vi "InstrumentCalibration - Sensor Setup (SubVI).vi"(8 "error in":errorcluster, 11 "Edit":string[](array[string])) -> (0 "error out":errorcluster)   [LabVIEW 2019]
uses:
  Controls/Sensor Setup - State.ctl
  Controls/Sensor Setup - Data Structure.ctl
  <vilib>/Analysis/NI_AALPro.lvlib
  Controls/FGV States.ctl
  Controls/Calibration - Data Structure.ctl
  Controls/eFGV States.ctl
  <vilib>/Utility/config.llb/NI_LVConfig.lvlib
  <vilib>/Utility/config.llb/Write Key (I32).vi
panel:
  in  "Status":u16(ring) items=["DISABLE", "ACTIVE"]
  in  "Decimal Place":i32=5
  in  "Close":bool
  in  "Load":bool
  in  "Save":bool
  in  "Tab":enum32{"Sensor", "Displacement"}(tab)
  in  "Serial No":string
  in  "Tab 2":enum32{"Direct Factor", "Multiple Point"}(tab)
  in  "Offset":dbl format="%#_5g"
  in  "Max Capacity [EU]":dbl format="%#_5g"
  in  "Maximum Voltage [V]":dbl format="%#_5g"
  in  "Table Control":string[][](table)
  in  "Calibrate":bool
  in  "Sensor Name":string
  in  "Sensor Port":T1(ring)
  in  "Unit":string
  out "Calibrated":dbl
  out "Raw (mV/V)":dbl format="%#_10f"
  out "Disp M":dbl
  in  "Zero":bool
  in  "Unit Disp":string caption="Unit"
  in  "Displacement":dbl
  in  "Calibrate Disp":bool
  out "Motor pulse":u64
  in  "Motor":T2(ring)
  # "1 (Unit) ="
  # "Pulse"
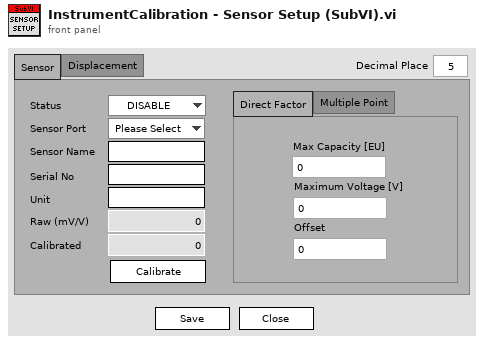
[diagram p1: front panel]
types:
  T1 = enum16{"Please Select", "LC 1", "LC 2", "LC 3", "LC 4", "LC 5", "LC 6", "LC 7", "LC 8", "TD 1", "TD 2", "TD 3", "TD 4", "TD 5", "TD 6", "TD 7", "TD 8", "TD 9", "TD 10", "TD 11", "TD 12"}
  T2 = enum16{"Please Select", "Motor 1", "Motor 2", "Motor 3", "Motor 4", "Motor 5", "Motor 6", "Motor 7", "Motor 8", "Motor 9"}
  T3 = typedef "Sensor Setup - State.ctl" = enum16{"Init", "Idle", "Save", "Close"}
  T4 = enum16{"open", "replace", "create", "open or create", "replace or create", "replace or create with confirmation"}
  T5 = typedef "Sensor Setup - State.ctl" = enum16{"Init", "Idle", "Read", "Calibrate", "Calibrate Disp", "Zeroing", "Zeroing Disp", "Save", "Save Calibration", "Load", "Load Calibration", "Update FGV", "Update GUI", "Close"}
  T6 = typedef "Sensor Setup - Data Structure.ctl" = cluster{"serialno":string, "Name":string, "Channel":string, "Slope":string, "Intercept":string, "Unit":string, "Decimal":string, "New?":bool, "Data":T7, "Port":string[], "IP":string[]}
  T7 = typedef "Calibration - Data Structure.ctl" = cluster{"Timeout":i32, "LC MC":dbl[], "TD MC":dbl[], "Motor Pulse":u64, "Disp M":dbl[], "LC Unit":string[], "Disp Unit":string[], "TD Unit":string[], "LC Name":string[], "TD Name":string[], "Machine":enum16{"Please Select", "Motor 1", "Motor 2", "Motor 3", "Motor 4", "Motor 5", "Motor 6", "Motor 7", "Motor 8", "Motor 9"}, "Sensor Port":enum16{"Please Select", "LC 1", "LC 2", "LC 3", "LC 4", "LC 5", "LC 6", "LC 7", "LC 8", "TD 1", "TD 2", "TD 3", "TD 4", "TD 5", "TD 6", "TD 7", "TD 8", "TD 9", "TD 10", "TD 11", "TD 12"}[]}
  T8 = typedef "FGV States.ctl" = enum16{"Read", "Write"}
  T9 = typedef "eFGV States.ctl" = enum16{"Init", "Read", "Write", "Exit"}
  T10 = cluster{"Zero":bool, "Machine Name":enum16{"Please Select", "Motor 1", "Motor 2", "Motor 3", "Motor 4", "Motor 5", "Motor 6", "Motor 7", "Motor 8", "Motor 9"}}
  T11 = enum16{"Please Select", "LC 1", "LC 2", "LC 3", "LC 4", "LC 5", "LC 6", "LC 7", "LC 8", "TD 1", "TD 2", "TD 3", "TD 4", "TD 5", "TD 6", "TD 7", "TD 8", "TD 9", "TD 10", "TD 11", "TD 12"}[]
  T12 = typedef "NI_LVConfig.lvlib/Config Data RefNum.ctl" = refnum<k1>
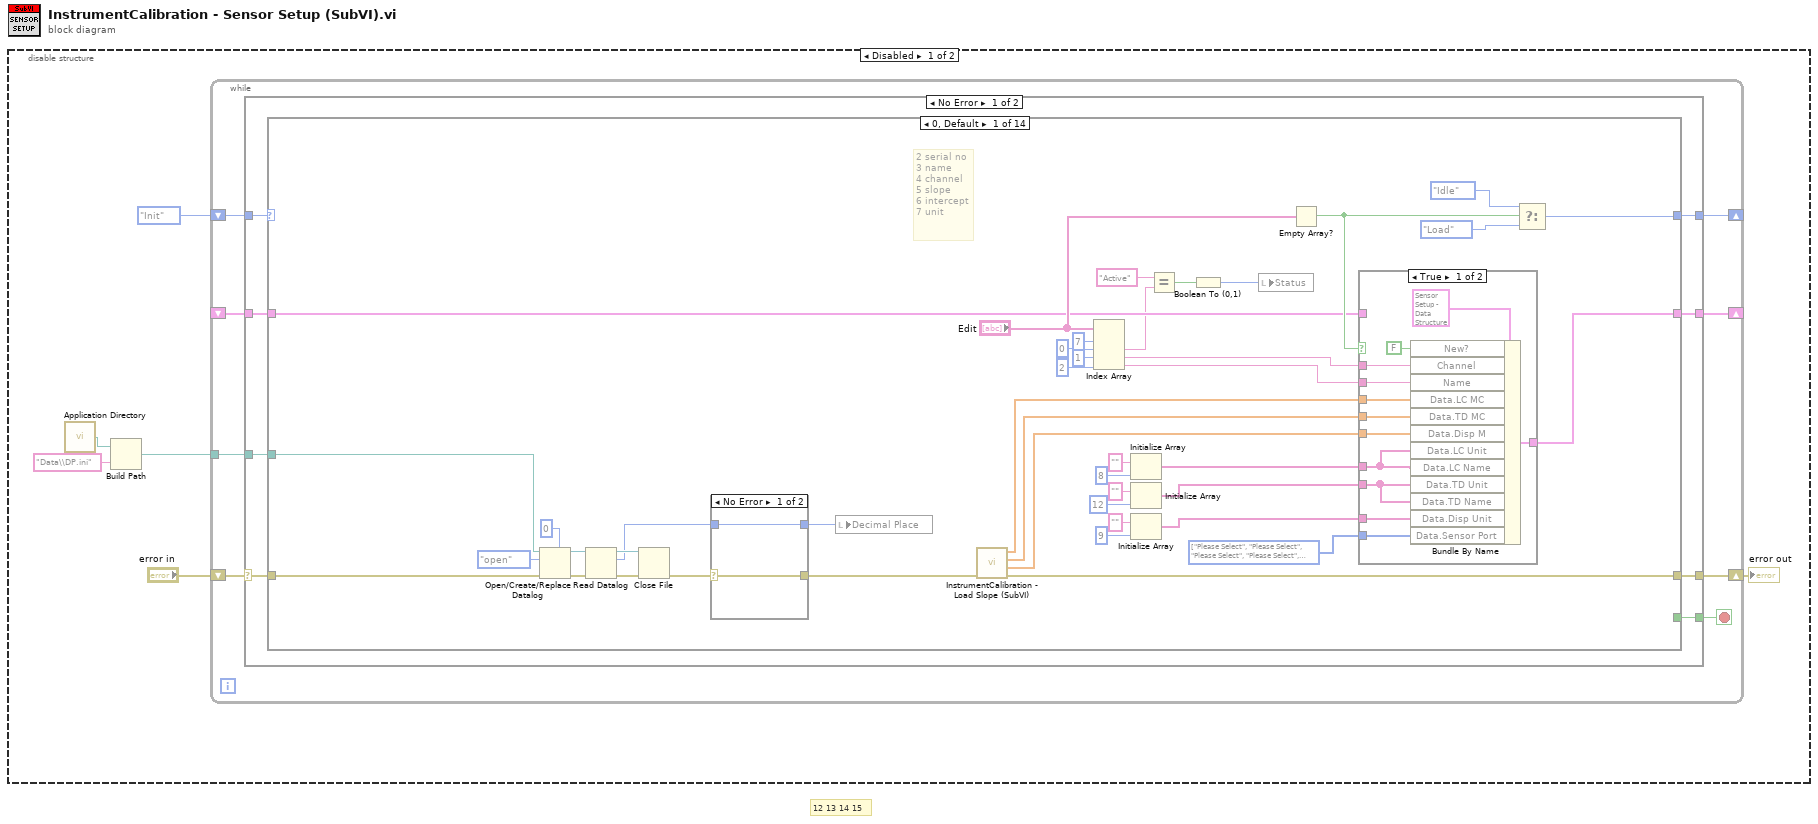
[diagram p0: block diagram]
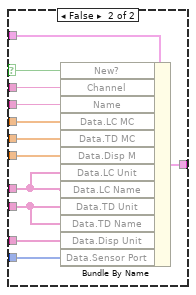
[diagram p2: hidden frame]
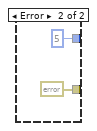
[diagram p3: hidden frame]
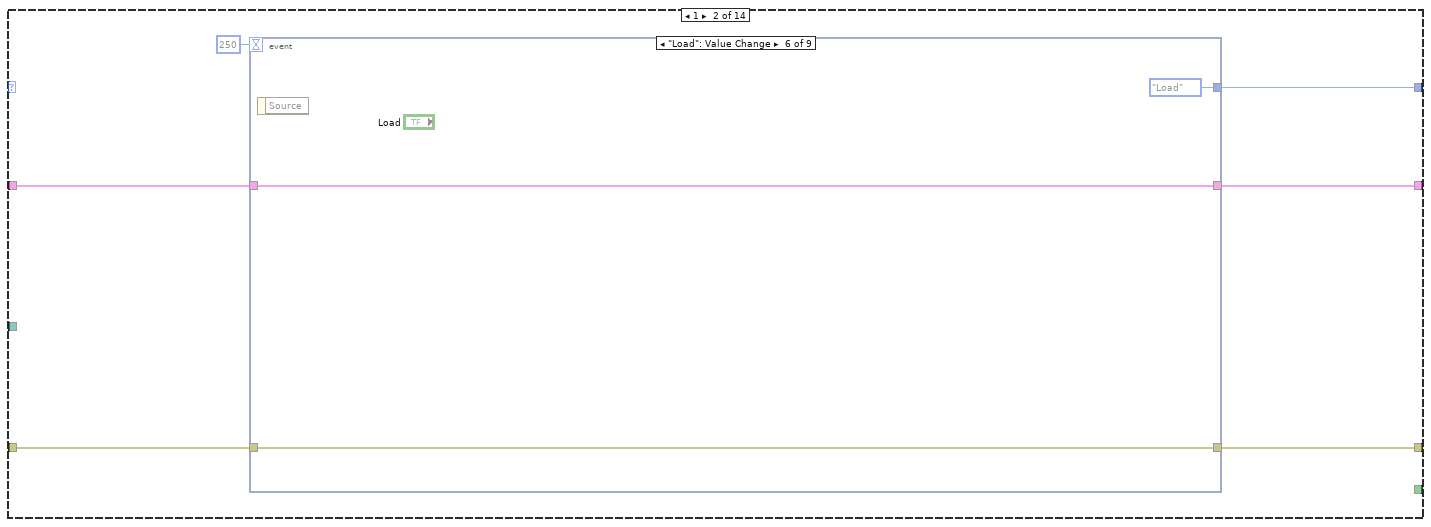
[diagram p4: hidden frame]
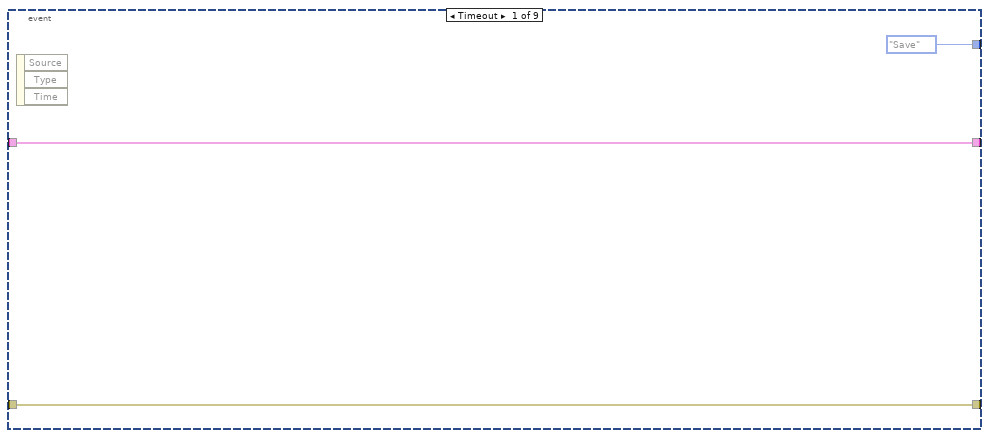
[diagram p5: hidden frame]
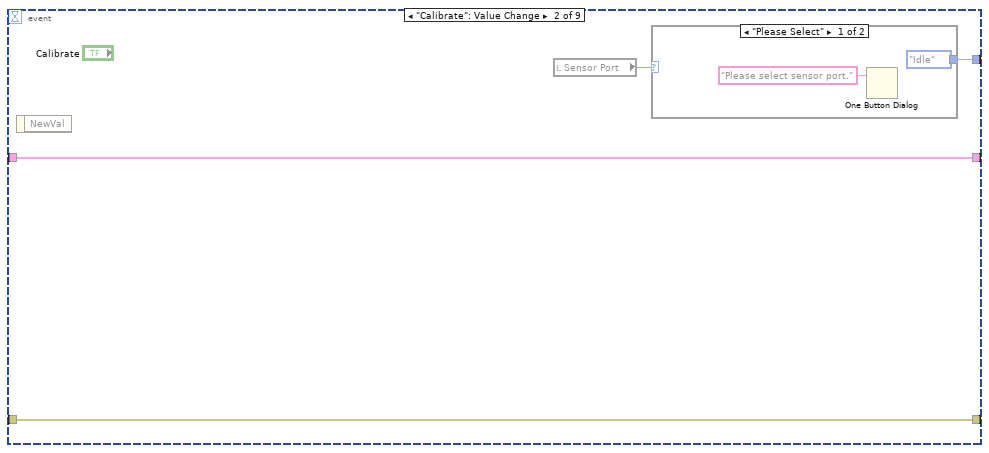
[diagram p6: hidden frame]
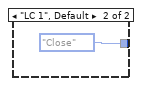
[diagram p7: hidden frame]
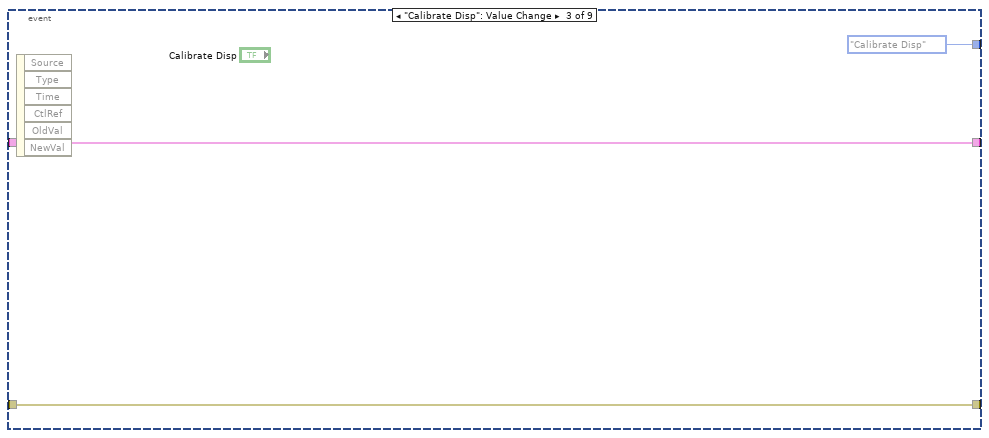
[diagram p8: hidden frame]
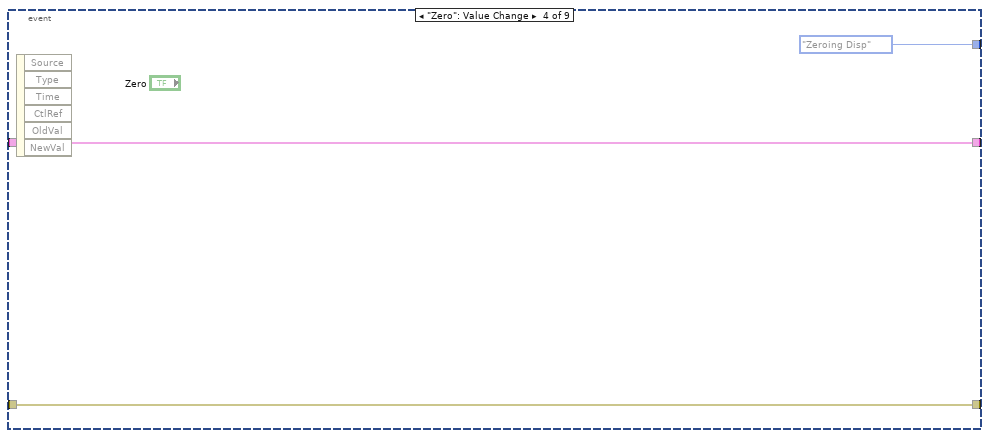
[diagram p9: hidden frame]
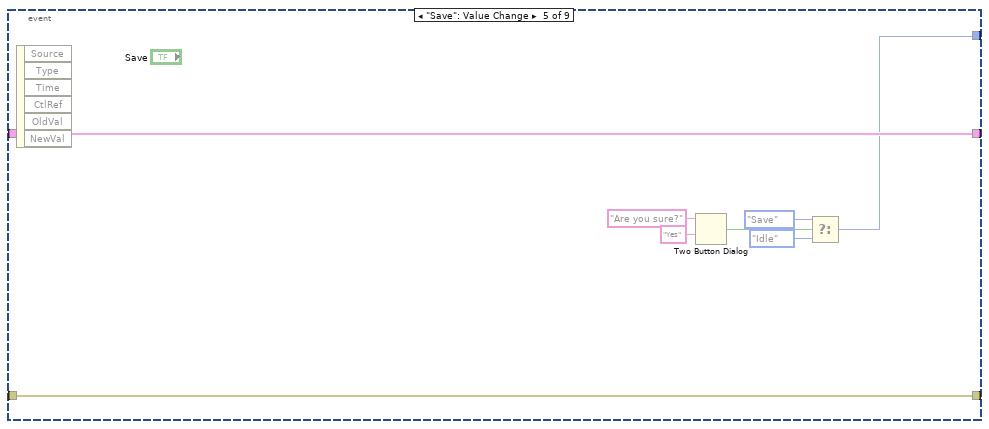
[diagram p10: hidden frame]
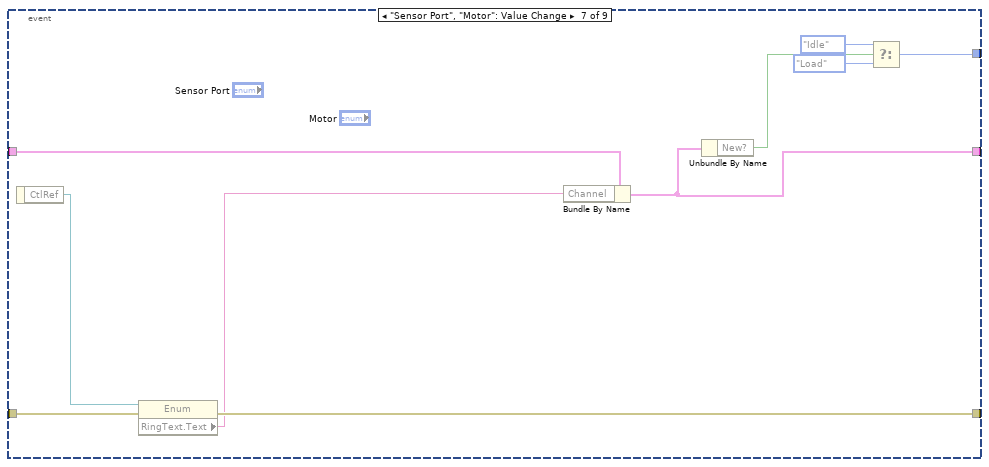
[diagram p11: hidden frame]
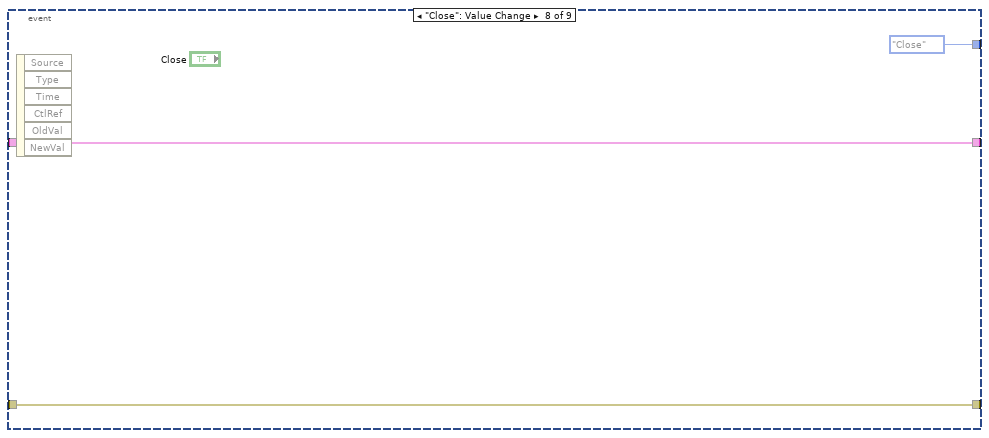
[diagram p12: hidden frame]
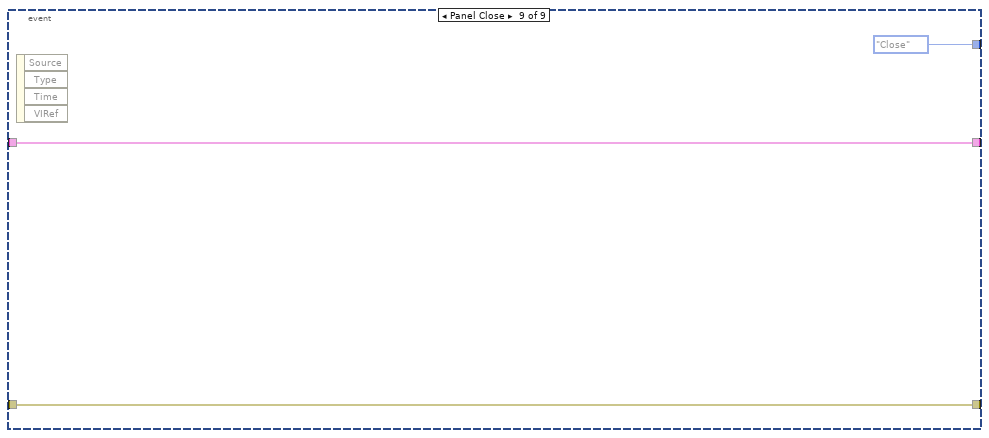
[diagram p13: hidden frame]
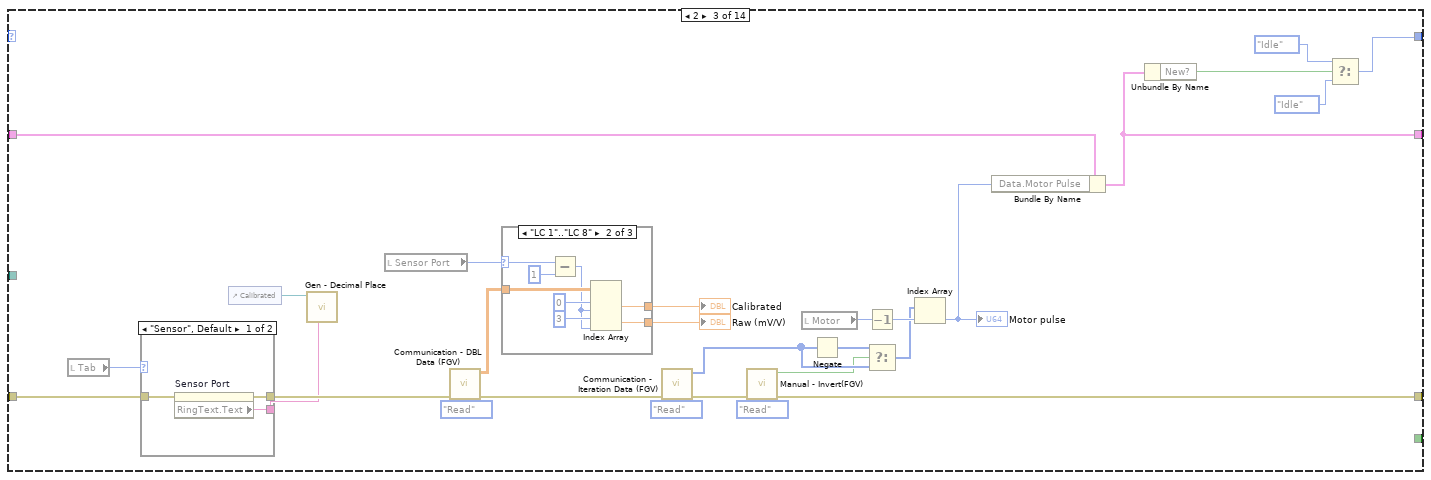
[diagram p14: hidden frame]
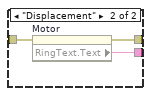
[diagram p15: hidden frame]
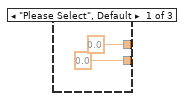
[diagram p16: hidden frame]
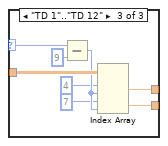
[diagram p17: hidden frame]
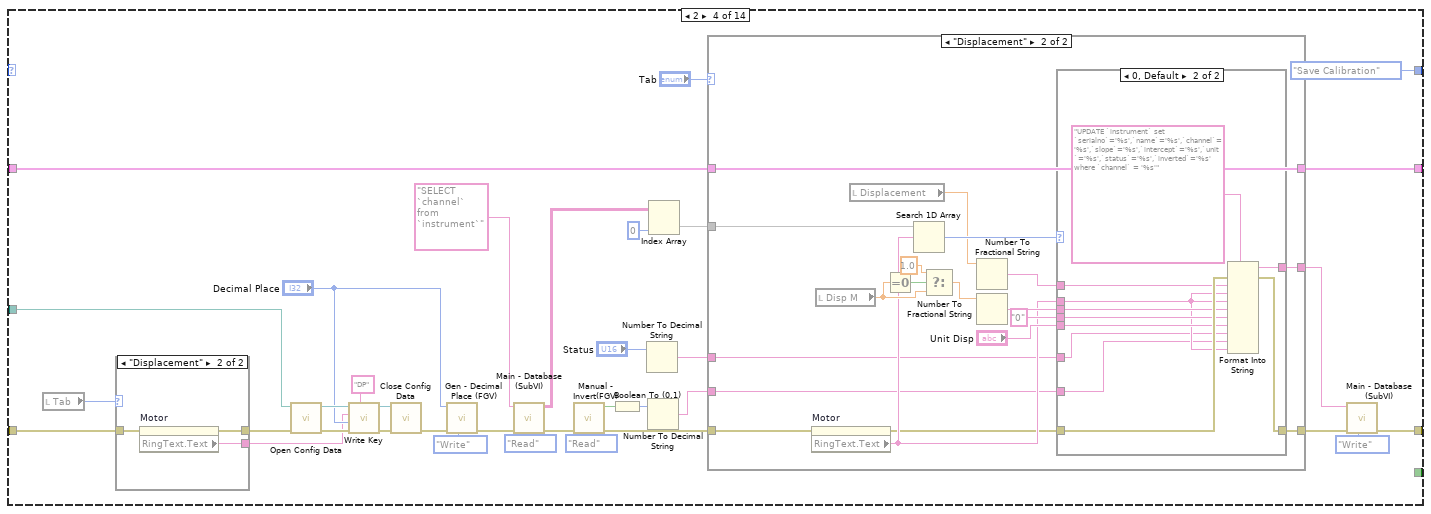
[diagram p18: hidden frame]
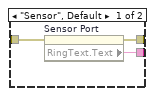
[diagram p19: hidden frame]
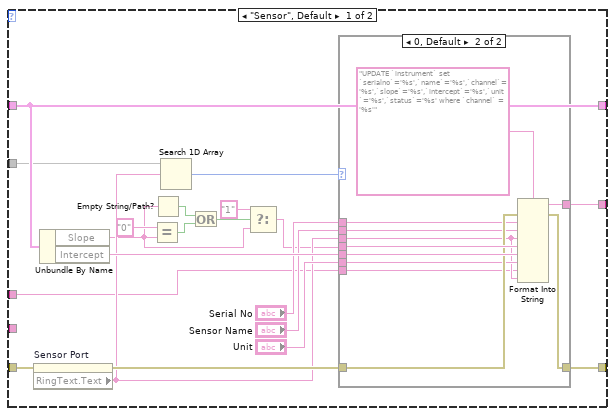
[diagram p20: hidden frame]
diagram:
  # "12 13 14 15"
  n1 = disable-structure shown="Disabled" {
    frame Disabled {
      n2 = call <vilib>:"Application Directory.vi"() -> ("Application Directory"=w3:path)
      n3 = Build Path(base path=w3, name or relative path="Data\\DP.ini") -> (appended path=w1:path)
      n4 = while {
        shift-right: [w13] -> _
        shift-left: Sensor_Setup_-_State."Init" -> [w14]
        shift-right: [w11] -> w4
        shift-left: "error in" -> [w12]
        shift-right: [w9] -> _
        shift-left: _ -> [w8]
        tunnel: w1 -> [w7]
        stop <- w10 stop-if-true
        n5 = case shown="No Error" w12 {
          selector: w12 -> [w19 w673]
          tunnel: w14 -> [w22 w669]
          tunnel: [w21 w669] -> w13
          tunnel: [w20 w672] -> w11
          tunnel: [w18 _] -> w10
          tunnel: [w17 w670] -> w9
          tunnel: w8 -> [w16 w670]
          tunnel: w7 -> [w15 _]
          frame No Error {
            n6 = case shown="0, Default" w22 {
              tunnel: [w60 w97 w159 Sensor_Setup_-_State."Save Calibration" Sensor_Setup_-_State."Load" Sensor_Setup_-_State."Load Calibration" Sensor_Setup_-_State."Update FGV" Sensor_Setup_-_State."Update GUI" Sensor_Setup_-_State."Idle" Sensor_Setup_-_State."Update FGV" Sensor_Setup_-_State."Idle" Sensor_Setup_-_State."Idle" Sensor_Setup_-_State."Close" Sensor_Setup_-_State."Idle"] -> w21
              tunnel: [w30 w99 w151 w225 w319 w367 w480 w526 w544 w570 w649 w652 w656 w659] -> w20
              tunnel: w19 -> [w42 w98 w146 w197 w323 w369 w476 w525 w544 w571 w649 w652 w656 w660]
              tunnel: [_ _ _ _ _ _ _ _ _ _ _ _ TRUE _] -> w18
              tunnel: [w65 w96 w161 w227 w321 w354 w481 w531 w538 w577 w640 w651 w653 w661] -> w17
              tunnel: w16 -> [w32 w95 w163 w228 w322 w353 w483 w531 w541 w565 w639 w651 w653 w661]
              tunnel: w15 -> [w41 _ _ w200 _ _ _ _ _ _ _ _ _ _]
              frame 0, Default {
                w52 = T11 [enum."Please Select", enum."Please Select", enum."Please Select", enum."Please Select", enum."Please Select", enum."Please Select", enum."Please Select", enum."Please Select", enum."Please Select"] items=["Please Select", "LC 1", "LC 2", "LC 3", "LC 4", "LC 5", "LC 6", "LC 7", "LC 8", "TD 1", "TD 2", "TD 3", "TD 4", "TD 5", "TD 6", "TD 7", "TD 8", "TD 9", "TD 10", "TD 11", "TD 12"] ("Sensor Port")
                # "2 serial no\n3 name\n4 channel\n5 slope\n6 intercept\n7 unit"
                n7 = Open/Create/Replace Datalog(5:0, 8:w42, 10:T4."open" ("operation (0:open)"), 11:w41) -> (0:w48:errorcluster, 3:w46:refnum<k1>)  [unwired: 2 in, 1 out]
                n8 = Read Datalog(4:w48, 7:w46) -> (0:w47:errorcluster, 2:w38:i32, 3:w45:refnum<k1>)  [unwired: 1 in]
                n9 = Close File(refnum=w45, error in=w47) -> (error out=w40:errorcluster)  [unwired: 1 out]
                n10 = case shown="No Error" w40 {
                  selector: w40 -> [w90 _]
                  tunnel: [w91 5] -> w39
                  tunnel: w38 -> [w91 _]
                  tunnel: [w90 errorcluster {"status"=FALSE, "code"=0, "source"=""} ("error IO")] -> w31
                  frame No Error {
                  }
                  frame Error {
                  }
                }
                n11 = local write "Decimal Place"(w39) -> ()
                n12 = call "InstrumentCalibration - Load Slope (SubVI).vi"("error in (no error)"=w31) -> ("error out"=w30:errorcluster, "Motor M"=w27:dbl[], "TD MC"=w28:dbl[], "LC MC"=w29:dbl[])  [unwired: 7 in]
                n13 = Index Array(array="Edit", index #1=7 ("index"), index #2=0 ("index"), index #3=1 ("index"), index #4=2 ("index")) -> (element #2=w26:string, element #3=w64:string, element #4=w63:string)  [unwired: 1 out]
                n14 = Initialize Array("" ("element"), 8 ("dimension size")) -> (w51:string[])
                n15 = Initialize Array("" ("element"), 12 ("dimension size")) -> (w50:string[])
                n16 = Initialize Array("" ("element"), 9 ("dimension size")) -> (w49:string[])
                n17 = Equal?(x="Active", y=w26) -> (x = y?=w24:bool)
                n18 = Boolean To (0,1)(Boolean=w24) -> (0, 1=w23:i16)
                n19 = local write "Status"(w23) -> ()
                n20 = Empty Array?(array="Edit") -> (empty?=w33:bool)
                n21 = case shown="True" w33 {
                  selector: w33 -> [_ w81]
                  tunnel: [w76 w89] -> w65
                  tunnel: w64 -> [w75 w88]
                  tunnel: w63 -> [w74 w87]
                  tunnel: w52 -> [w73 w86]
                  tunnel: w29 -> [w72 w85]
                  tunnel: w28 -> [w71 w84]
                  tunnel: w27 -> [w70 w83]
                  tunnel: w51 -> [w68 w80]
                  tunnel: w50 -> [w67 w79]
                  tunnel: w49 -> [w69 w82]
                  tunnel: w32 -> [_ w78]
                  frame True {
                    n22 = Bundle By Name(cluster=T6 {"serialno"="", "Name"="", "Channel"="", "Slope"="", "Intercept"="", "Unit"="", "Decimal"="", "New?"=FALSE, "Data"={"Timeout"=-1, "LC MC"=[], "TD MC"=[], "Motor Pulse"=0, "Disp M"=[], "LC Unit"=[], "Disp Unit"=[], "TD Unit"=[], "LC Name"=[], "TD Name"=[], "Machine"=enum."Please Select", "Sensor Port"=[]}, "Port"=[], "IP"=[]}, "New?"=FALSE, "Channel"=w75, "Name"=w74, "Data.LC MC"=w72, "Data.TD MC"=w71, "Data.Disp M"=w70, "Data.LC Unit"=w68, "Data.LC Name"=w68, "Data.TD Unit"=w67, "Data.TD Name"=w67, "Data.Disp Unit"=w69, "Data.Sensor Port"=w73) -> (w76:T6)
                  }
                  frame False {
                    n23 = Bundle By Name(cluster=w78, "New?"=w81, "Channel"=w88, "Name"=w87, "Data.LC MC"=w85, "Data.TD MC"=w84, "Data.Disp M"=w83, "Data.LC Unit"=w80, "Data.LC Name"=w80, "Data.TD Unit"=w79, "Data.TD Name"=w79, "Data.Disp Unit"=w82, "Data.Sensor Port"=w86) -> (w89:T6)
                  }
                }
                n24 = Select(t=Sensor_Setup_-_State."Idle", s=w33, f=Sensor_Setup_-_State."Load") -> (s? t:f=w60:u16)
              }
              frame 1 {
                n25 = event shown="[5] \"Load\": Value Change" {
                  selector: _ -> [_ _ _ _ _ _ _ _ _]
                  dyn-events: _ -> [_ _ _ _ _ _ _ _ _]
                  timeout: 250 -> [_ _ _ _ _ _ _ _ _]
                  tunnel: [w102 w106 w112 w115 w123 w126 w134 w139 w142] -> w99
                  tunnel: w98 -> [w102 w106 w112 w115 w123 w126 w133 w139 w142]
                  tunnel: [Sensor_Setup_-_State."Save" w105 Sensor_Setup_-_State."Calibrate Disp" Sensor_Setup_-_State."Zeroing Disp" w117 Sensor_Setup_-_State."Load" w128 Sensor_Setup_-_State."Close" Sensor_Setup_-_State."Close"] -> w97
                  tunnel: [w100 w104 w110 w113 w122 w124 w131 w138 w141] -> w96
                  tunnel: w95 -> [w100 w104 w110 w113 w122 w124 w136 w138 w141]
                  event Timeout {
                    n26 = event-data() -> ()  [unwired: 1 in, 3 out]
                  }
                  event "Calibrate": Value Change {
                    n27 = event-data() -> ()  [unwired: 1 in, 1 out]
                    n28 = local read "Sensor Port"() -> (w103:T1)
                    n29 = case shown="\"Please Select\"" w103 {
                      tunnel: [Sensor_Setup_-_State."Idle" Sensor_Setup_-_State."Close"] -> w105
                      frame "Please Select" {
                        n30 = One Button Dialog(message="Please select sensor port.") -> ()  [unwired: 1 in, 1 out]
                      }
                      frame "LC 1", Default {
                      }
                    }
                  }
                  event "Calibrate Disp": Value Change {
                    n31 = event-data() -> ()  [unwired: 1 in, 6 out]
                  }
                  event "Zero": Value Change {
                    n32 = event-data() -> ()  [unwired: 1 in, 6 out]
                  }
                  event "Save": Value Change {
                    n33 = event-data() -> ()  [unwired: 1 in, 6 out]
                    n34 = Two Button Dialog(message="Are you sure?", 2:"Yes" ("T button name (\"OK\")")) -> (T button?=w119:bool)  [unwired: 1 in]
                    n35 = Select(t=Sensor_Setup_-_State."Save", s=w119, f=Sensor_Setup_-_State."Idle") -> (s? t:f=w117:T3)
                  }
                  event "Load": Value Change {
                    n36 = event-data() -> ()  [unwired: 1 in, 1 out]
                  }
                  event "Sensor Port", "Motor": Value Change {
                    n37 = event-data() -> ("CtlRef"=w135:refnum<vi>)  [unwired: 1 in]
                    n38 = property class="Enum"(reference=w135, error in=w133) -> (error out=w134:errorcluster, "RingText.Text"=w132:string)  [unwired: 1 out]
                    n39 = Bundle By Name(cluster=w136, "Channel"=w132) -> (w131:T6)
                    n40 = Unbundle By Name(w131) -> ("New?"=w130:bool)
                    n41 = Select(t=Sensor_Setup_-_State."Idle", s=w130, f=Sensor_Setup_-_State."Load") -> (s? t:f=w128:u16)
                  }
                  event "Close": Value Change {
                    n42 = event-data() -> ()  [unwired: 1 in, 6 out]
                  }
                  event Panel Close {
                    n43 = event-data() -> ()  [unwired: 1 in, 4 out]
                  }
                }
              }
              frame 2 {
                n44 = local read "Tab"() -> (w147:enum32{"Sensor", "Displacement"})
                n45 = case shown="\"Sensor\", Default" w147 {
                  tunnel: [w172 w176] -> w145
                  tunnel: w146 -> [w173 w175]
                  tunnel: [w171 w174] -> w144
                  frame "Sensor", Default {
                    n46 = property on="Sensor Port" class="Enum (strict)"(error in=w173) -> (error out=w172:errorcluster, "RingText.Text"=w171:string)  [unwired: 1 in, 1 out]
                  }
                  frame "Displacement" {
                    n47 = property on="Motor" class="Enum (strict)"(error in=w175) -> (error out=w176:errorcluster, "RingText.Text"=w174:string)  [unwired: 1 in, 1 out]
                  }
                }
                n48 = control-ref of="Calibrated"() -> (w143:refnum<vi>)
                n49 = call "Gen - Decimal Place.vi"(7:w144, "DigNum Refnum"=w143) -> ()  [unwired: 10 in]
                n50 = local read "Sensor Port"() -> (w148:T1)
                n51 = call "Communication - DBL Data (FGV).vi"("Action"=FGV_States."Read", "error in (no error)"=w145) -> ("error out"=w152:errorcluster, "DBL SV Out"=w169:dbl[][])  [unwired: 8 in]
                n52 = case shown="\"LC 1\"..\"LC 8\"" w148 {
                  selector: w148 -> [_ w181 w191]
                  tunnel: w169 -> [_ w186 w194]
                  tunnel: [0.0 ("shared variable refnum in") w185 w193] -> w168
                  tunnel: [0.0 ("shared variable refnum in") w184 w192] -> w167
                  frame "Please Select", Default {
                  }
                  frame "LC 1".."LC 8" {
                    n53 = Subtract(x=w181, y=1 ("disabled index (col)")) -> (x-y=w180:i32)
                    n54 = Index Array(array=w186, index (row) #1=0 ("disabled index (col)"), index (col) #1=w180, index (row) #2=3 ("index (col)"), index (col) #2=w180) -> (element #1=w185:dbl, element #2=w184:dbl)
                  }
                  frame "TD 1".."TD 12" {
                    n55 = Subtract(x=w191, y=9 ("disabled index (col)")) -> (x-y=w189:i32)
                    n56 = Index Array(array=w194, index (row) #1=4 ("disabled index (col)"), index (col) #1=w189, index (row) #2=7 ("index (col)"), index (col) #2=w189) -> (element #1=w193:dbl, element #2=w192:dbl)
                  }
                }
                "Raw (mV/V)" <- w167
                "Calibrated" <- w168
                n57 = call "Communication - Iteration Data (FGV).vi"("Action"=FGV_States."Read", "error in (no error)"=w152) -> ("error out"=w150:errorcluster, "Iteration SV Out"=w155:i64[])  [unwired: 8 in]
                n58 = call "Manual - Invert(FGV).vi"("Action"=FGV_States."Read", "error in (no error)"=w150) -> ("error out"=w151:errorcluster, "invert out"=w149:bool)  [unwired: 8 in]
                n59 = local read "Motor"() -> (w165:T2)
                n60 = Negate(x=w155) -> (-x=w156:i64[])
                n61 = Decrement(x=w165) -> (x-1=w166:T2)
                n62 = Select(t=w156, s=w149, f=w155) -> (s? t:f=w154:i64[])
                n63 = Index Array(array=w154, index=w166) -> (element=w162:i64)
                "Motor pulse" <- w162
                n64 = Bundle By Name(cluster=w163, "Data.Motor Pulse"=w162) -> (w161:T6)
                n65 = Unbundle By Name(w161) -> ("New?"=w160:bool)
                n66 = Select(t=Sensor_Setup_-_State."Idle", s=w160, f=Sensor_Setup_-_State."Idle") -> (s? t:f=w159:T3)
              }
              frame 2 {
                n67 = local read "Tab"() -> (w195:enum32{"Sensor", "Displacement"})
                n68 = case shown="\"Displacement\"" w195 {
                  tunnel: [w231 w235] -> w198
                  tunnel: w197 -> [w232 w234]
                  tunnel: [w230 w233] -> w196
                  frame "Sensor", Default {
                    n69 = property on="Sensor Port" class="Enum (strict)"(error in=w232) -> (error out=w231:errorcluster, "RingText.Text"=w230:string)  [unwired: 1 in, 1 out]
                  }
                  frame "Displacement" {
                    n70 = property on="Motor" class="Enum (strict)"(error in=w234) -> (error out=w235:errorcluster, "RingText.Text"=w233:string)  [unwired: 1 in, 1 out]
                  }
                }
                n71 = call <vilib>:"Open Config Data.vi"("error in (no error)"=w198, "configuration file path"=w200) -> ("error out"=w205:errorcluster, "refnum"=w203:T12)  [unwired: 7 in, 1 out]
                n72 = call-poly <vilib>:"Write Key.vi"("section"="DP", "error in (no error)"=w205, "value"="Decimal Place", "key"=w196, "refnum"=w203) -> ("error out"=w206:errorcluster, "refnum out"=w204:T12)  [unwired: 4 in, 1 out]
                n73 = call <vilib>:"Close Config Data.vi"("error in (no error)"=w206, "refnum"=w204) -> ("error out"=w201:errorcluster)  [unwired: 8 in, 1 out]
                n74 = call "Gen - Decimal Place (FGV).vi"("Action"=FGV_States."Write", "error In"=w201, "Ch1"="Decimal Place") -> ("error out"=w210:errorcluster)  [unwired: 6 in, 2 out]
                n75 = call "Main - Database (SubVI).vi"("Enum"=FGV_States."Read", "error in (no error)"=w210, "SQL query"="SELECT `channel` from `instrument`") -> ("error out"=w215:errorcluster, "data"=w219:string[][])  [unwired: 7 in]
                n76 = call "Manual - Invert(FGV).vi"("Action"=FGV_States."Read", "error in (no error)"=w215) -> ("error out"=w214:errorcluster, "invert out"=w213:bool)  [unwired: 8 in]
                n77 = Boolean To (0,1)(Boolean=w213) -> (0, 1=w209:i16)
                n78 = Number To Decimal String(number="Status") -> (decimal integer string=w207:string)  [unwired: 1 in]
                n79 = Number To Decimal String(number=w209) -> (decimal integer string=w212:string)  [unwired: 1 in]
                n80 = Index Array(array=w219, index (col)=0 ("disabled index (col)")) -> (element=w218:string[])  [unwired: 1 in]
                n81 = case shown="\"Displacement\"" "Tab" {
                  tunnel: w228 -> [w255 w296]
                  tunnel: [w255 w296] -> w227
                  tunnel: w214 -> [w252 w295]
                  tunnel: [w248 w291] -> w223
                  tunnel: [w247 w290] -> w222
                  tunnel: w218 -> [w246 w289]
                  tunnel: w212 -> [_ w279]
                  tunnel: w207 -> [w236 w278]
                  frame "Sensor", Default {
                    n82 = property on="Sensor Port" class="Enum (strict)"(error in=w252) -> (error out=w253:errorcluster, "RingText.Text"=w245:string)  [unwired: 1 in, 1 out]
                    n83 = Unbundle By Name(w255) -> ("Slope"=w239:string, "Intercept"=w254:string)
                    n84 = Equal?(x="0", y=w239) -> (x = y?=w241:bool)
                    n85 = Empty String/Path?(string/path=w239) -> (empty?=w242:bool)
                    n86 = Search 1D Array(1D array=w246, element=w245) -> (index of element=w244:i32)  [unwired: 1 in]
                    n87 = Or(x=w242, y=w241) -> (x .or. y?=w240:bool)
                    n88 = Select(t="1", s=w240, f=w239) -> (s? t:f=w237:string)
                    n89 = case shown="0, Default" w244 {
                      tunnel: w237 -> [w265 w277]
                      tunnel: w254 -> [w264 w276]
                      tunnel: w253 -> [w263 w275]
                      tunnel: "Unit" -> [w262 w274]
                      tunnel: "Serial No" -> [w261 w273]
                      tunnel: "Sensor Name" -> [w260 w272]
                      tunnel: w245 -> [w259 w268]
                      tunnel: [w258 w271] -> w248
                      tunnel: [w257 w270] -> w247
                      tunnel: w236 -> [w256 w267]
                      frame -1 {
                        n90 = Format Into String(format string="INSERT INTO `instrument`  (`serialno`,`name`,`channel`,`slope`,`intercept`,`unit`,`status`) VALUES ('%s','%s','%s','%s','%s','%s','%s')" ("SQL query"), error in=w263, w261, w260, w259, w265, w264, w262, w256) -> (resulting string=w257:string, error out=w258:errorcluster)  [unwired: 1 in]
                      }
                      frame 0, Default {
                        n91 = Format Into String(format string="UPDATE `instrument` set `serialno`='%s',`name`='%s',`channel`='%s',`slope`='%s',`intercept`='%s',`unit`='%s',`status`='%s' where `channel` = '%s'" ("SQL query"), error in=w275, w273, w272, w268, w277, w276, w274, w267, w268) -> (resulting string=w270:string, error out=w271:errorcluster)  [unwired: 1 in]
                      }
                    }
                  }
                  frame "Displacement" {
                    n92 = property on="Motor" class="Enum (strict)"(error in=w295) -> (error out=w280:errorcluster, "RingText.Text"=w281:string)  [unwired: 1 in, 1 out]
                    n93 = local read "Disp M"() -> (w285:dbl)
                    n94 = local read "Displacement"() -> (w283:dbl)
                    n95 = Equal To 0?(x=w285) -> (x = 0?=w287:bool)
                    n96 = Search 1D Array(1D array=w289, element=w281) -> (index of element=w288:i32)  [unwired: 1 in]
                    n97 = Select(t=1.0, s=w287, f=w285) -> (s? t:f=w284:dbl)
                    n98 = Number To Fractional String(number=w283) -> (F-format string=w282:string)  [unwired: 3 in]
                    n99 = Number To Fractional String(number=w284) -> (F-format string=w292:string)  [unwired: 3 in]
                    n100 = case shown="0, Default" w288 {
                      tunnel: w280 -> [w306 w317]
                      tunnel: w281 -> [w300 w310]
                      tunnel: "Unit Disp" -> [w305 w316]
                      tunnel: "0" -> [w304 w315]
                      tunnel: w292 -> [w303 w314]
                      tunnel: [w302 w313] -> w291
                      tunnel: [w301 w312] -> w290
                      tunnel: w282 -> [w299 w311]
                      tunnel: w279 -> [w297 w309]
                      tunnel: w278 -> [w298 w308]
                      frame -1 {
                        n101 = Format Into String(format string="INSERT INTO `instrument`  (`serialno`,`name`,`channel`,`slope`,`intercept`,`unit`,`status`,`inverted`) VALUES ('%s','%s','%s','%s','%s','%s','%s','%s')" ("SQL query"), error in=w306, w299, w300, w300, w303, w304, w305, w298, w297) -> (resulting string=w301:string, error out=w302:errorcluster)  [unwired: 1 in]
                      }
                      frame 0, Default {
                        n102 = Format Into String(format string="UPDATE `instrument` set `serialno`='%s',`name`='%s',`channel`='%s',`slope`='%s',`intercept`='%s',`unit`='%s',`status`='%s',`inverted`='%s' where `channel` = '%s'" ("SQL query"), error in=w317, w311, w310, w310, w314, w315, w316, w308, w309, w310) -> (resulting string=w312:string, error out=w313:errorcluster)  [unwired: 1 in]
                      }
                    }
                  }
                }
                n103 = call "Main - Database (SubVI).vi"("Enum"=FGV_States."Write", "error in (no error)"=w223, "SQL query"=w222) -> ("error out"=w225:errorcluster)  [unwired: 7 in, 1 out]
              }
              frame 3 {
                n104 = local read "Tab"() -> (w320:enum32{"Sensor", "Displacement"})
                n105 = case shown="\"Sensor\"" w320 {
                  tunnel: w322 -> [w346 w352]
                  tunnel: [w346 w352] -> w321
                  tunnel: w323 -> [w344 w351]
                  tunnel: [w339 w351] -> w319
                  frame "Sensor" {
                    n106 = local read "Table Control"() -> (w325:string[][])
                    n107 = for {
                      tunnel: w325 -> [w347] mode=indexing
                      tunnel: [w348] -> w327 mode=indexing
                      n108 = Array To Spreadsheet String(delimiter (Tab)=",,", array=w347, 3:"" ("format string")) -> (spreadsheet string=w348:string)
                    }
                    n109 = Array To Spreadsheet String(delimiter (Tab)="||", array=w327, 3:"" ("format string")) -> (spreadsheet string=w326:string)
                    n110 = local read "Maximum Voltage [V]"() -> (w332:dbl)
                    n111 = local read "Max Capacity [EU]"() -> (w333:dbl)
                    n112 = property on="Sensor Port" class="Enum (strict)"(error in=w344) -> (error out=w345:errorcluster, "RingText.Text"=w343:string)  [unwired: 1 in, 1 out]
                    n113 = local read "Tab 2"() -> (w337:enum32{"Direct Factor", "Multiple Point"})
                    n114 = Number To Fractional String(number=w333, precision (6)=i16 6) -> (F-format string=w331:string)  [unwired: 2 in]
                    n115 = Number To Fractional String(number=w332, precision (6)=i16 6) -> (F-format string=w330:string)  [unwired: 2 in]
                    n116 = Number To Decimal String(number=w337) -> (decimal integer string=w336:string)  [unwired: 1 in]
                    n117 = Format Into String(format string="UPDATE `instrument` set `tab`='%s',`max_cap`='%s',`max_v`='%s',`multipoint`='%s'  where `channel` = '%s'" ("SQL query"), error in=w345, w336, w331, w330, w326, w343) -> (resulting string=w338:string, error out=w340:errorcluster)  [unwired: 1 in]
                    n118 = call "Main - Database (SubVI).vi"("Enum"=FGV_States."Write", "error in (no error)"=w340, "SQL query"=w338) -> ("error out"=w339:errorcluster)  [unwired: 7 in, 1 out]
                  }
                  frame "Displacement", Default {
                  }
                }
              }
              frame 1 {
                n119 = Unbundle By Name(w353) -> ("Channel"=w366:string)
                n120 = Search and Replace String(input string=w366, search string="Motor", error in=w369) -> (number of replacements=w368:i32, error out=w370:errorcluster)  [unwired: 5 in, 2 out]
                n121 = case shown="..0" w368 {
                  tunnel: [w468 w473] -> w364
                  tunnel: w370 -> [w467 w474]
                  tunnel: w366 -> [w464 w469]
                  tunnel: [w464 w469] -> w358
                  tunnel: [enum32{"Sensor", "Displacement"}."Sensor" ("Tab") enum32{"Sensor", "Displacement"}."Displacement" ("Tab")] -> w356
                  frame ..0 {
                    n122 = property on="Sensor Port" class="Enum (strict)"(error in=w467) -> (error out=w468:errorcluster, "Strings []"=w466:string[])  [unwired: 1 in, 1 out]
                    n123 = Search 1D Array(1D array=w466, element=w464) -> (index of element=w465:i32)  [unwired: 1 in]
                    n124 = local write "Sensor Port"(w465) -> ()
                  }
                  frame 1.. {
                    n125 = property on="Motor" class="Enum (strict)"(error in=w474) -> (error out=w473:errorcluster, "Strings []"=w471:string[])  [unwired: 1 in, 1 out]
                    n126 = Search 1D Array(1D array=w471, element=w469) -> (index of element=w472:i32)  [unwired: 1 in]
                    n127 = local write "Motor"(w472) -> ()
                  }
                }
                n128 = Format Into String(format string="SELECT * from `instrument` where `channel` ='%s'" ("SQL query"), error in=w364, w358) -> (resulting string=w361:string, error out=w363:errorcluster)  [unwired: 1 in]
                n129 = local write "Tab"(w356) -> ()
                n130 = call "Main - Database (SubVI).vi"("Enum"=FGV_States."Read", "error in (no error)"=w363, "SQL query"=w361) -> ("error out"=w355:errorcluster, "data"=w360:string[][])  [unwired: 7 in]
                n131 = Index Array(array=w360, index (row)=0) -> (element=w357:string[])  [unwired: 1 in]
                n132 = case shown="\"Sensor\", Default" w356 {
                  tunnel: w357 -> [w397 w462]
                  tunnel: [w388 w461] -> w367
                  tunnel: w355 -> [w389 w461]
                  tunnel: w353 -> [w393 w454]
                  tunnel: w353 -> [w390 w453]
                  tunnel: [w387 w452] -> w354
                  frame "Sensor", Default {
                    n133 = Index Array(array=w397, index #1=2 ("index"), index #2=3 ("index"), index #3=5 ("index"), index #4=6 ("index"), index #5=7 ("index"), index #6=11 ("index")) -> (element #1=w386:string, element #2=w385:string, element #3=w382:string, element #4=w381:string, element #5=w384:string, element #6=w374:string)
                    n134 = local read "Sensor Port"() -> (w383:T1)
                    n135 = Decimal String To Number(string=w374) -> (number=w373:i32)  [unwired: 2 in, 1 out]
                    n136 = Fract/Exp String To Number(string=w382) -> (number=w380:dbl)  [unwired: 3 in, 1 out]
                    n137 = Fract/Exp String To Number(string=w381) -> (number=w379:dbl)  [unwired: 3 in, 1 out]
                    n138 = case shown="\"TD 1\"..\"TD 12\"" w383 {
                      selector: w383 -> [_ w416 w438]
                      tunnel: w393 -> [w402 w422 w443]
                      tunnel: w390 -> [_ w421 w442]
                      tunnel: w389 -> [w398 w420 w441]
                      tunnel: [w398 w420 w441] -> w388
                      tunnel: [w402 w419 w440] -> w387
                      tunnel: w386 -> [_ w405 w423]
                      tunnel: w385 -> [_ w404 w428]
                      tunnel: w384 -> [_ w403 w429]
                      tunnel: w380 -> [_ w408 w436]
                      tunnel: w379 -> [_ w407 w435]
                      tunnel: ["" ("Value") w405 w423] -> w378
                      tunnel: ["" ("Value") w404 w428] -> w377
                      tunnel: ["" ("Value") w403 w429] -> w376
                      frame "Please Select", Default {
                      }
                      frame "LC 1".."LC 8" {
                        n139 = Decrement(x=w416) -> (x-1=w411:T1)
                        n140 = Unbundle By Name(w421) -> ("Data.LC MC"=w418:dbl[], "Data.LC Unit"=w413:string[], "Data.LC Name"=w410:string[])
                        n141 = Multiply(x=w411, y=2) -> (x*y=w415:i32)
                        n142 = Increment(x=w415) -> (x+1=w414:i32)
                        n143 = Replace Array Subset(array=w418, new element #1=w408, index #1=w415, new element #2=w407, index #2=w414) -> (w406:dbl[])
                        n144 = Replace Array Subset(array=w413, new element=w403, index=w411) -> (w412:string[])
                        n145 = Replace Array Subset(array=w410, new element=w404, index=w411) -> (w409:string[])
                        n146 = Bundle By Name(cluster=w422, "Data.LC MC"=w406, "Data.LC Unit"=w412, "Data.LC Name"=w409, "serialno"=w405) -> (w419:T6)
                      }
                      frame "TD 1".."TD 12" {
                        n147 = Unbundle By Name(w442) -> ("Data.TD MC"=w439:dbl[], "Data.TD Unit"=w433:string[], "Data.TD Name"=w432:string[])
                        n148 = Subtract(x=w438, y=9) -> (x-y=w424:i32)
                        n149 = Multiply(x=w424, y=2) -> (x*y=w426:i32)
                        n150 = Increment(x=w426) -> (x+1=w425:i32)
                        n151 = Replace Array Subset(array=w439, new element #1=w436, index #1=w426, new element #2=w435, index #2=w425) -> (w434:dbl[])
                        n152 = Replace Array Subset(array=w433, new element=w429, index=w424) -> (w430:string[])
                        n153 = Replace Array Subset(array=w432, new element=w428, index=w424) -> (w431:string[])
                        n154 = Bundle By Name(cluster=w443, "Data.TD MC"=w434, "Data.TD Unit"=w430, "Data.TD Name"=w431, "serialno"=w423) -> (w440:T6)
                      }
                    }
                    n155 = local write "Status"(w373) -> ()
                    n156 = local write "Serial No"(w378) -> ()
                    n157 = local write "Sensor Name"(w377) -> ()
                    n158 = local write "Unit"(w376) -> ()
                  }
                  frame "Displacement" {
                    n159 = Index Array(array=w462, index #1=2 ("index"), index #2=5 ("index"), index #3=7 ("index")) -> (element #1=w457:string, element #2=w455:string, element #3=w445:string)
                    n160 = Unbundle By Name(w453) -> ("Data.Disp M"=w451:dbl[], "Data.Disp Unit"=w447:string[])
                    n161 = local read "Motor"() -> (w450:T2)
                    n162 = Fract/Exp String To Number(string=w457) -> (number=w456:dbl)  [unwired: 3 in, 1 out]
                    n163 = Fract/Exp String To Number(string=w455) -> (number=w449:dbl)  [unwired: 3 in, 1 out]
                    n164 = Decrement(x=w450) -> (x-1=w446:T2)
                    n165 = Replace Array Subset(array=w451, new element=w449, index=w446) -> (w448:dbl[])
                    n166 = Replace Array Subset(array=w447, new element=w445, index=w446) -> (w444:string[])
                    n167 = Bundle By Name(cluster=w454, "Data.Disp M"=w448, "Data.Disp Unit"=w444) -> (w452:T6)
                    n168 = local write "Displacement"(w456) -> ()
                    n169 = local write "Disp M"(w449) -> ()
                    n170 = local write "Unit Disp"(w445) -> ()
                  }
                }
              }
              frame 2 {
                n171 = Unbundle By Name(w483) -> ("Channel"=w475:string)
                n172 = local read "Tab"() -> (w482:enum32{"Sensor", "Displacement"})
                n173 = call "Gen - Decimal Place (FGV).vi"(6:w475, "Action"=FGV_States."Read", "error In"=w476) -> ("error out"=w477:errorcluster, "Ch2 out"=w479:u8)  [unwired: 6 in, 1 out]
                n174 = local write "Decimal Place"(w479) -> ()
                n175 = case shown="\"Sensor\", Default" w482 {
                  tunnel: w477 -> [w509 w521]
                  tunnel: w483 -> [w503 w522]
                  tunnel: [w503 w522] -> w481
                  tunnel: [w492 w521] -> w480
                  tunnel: w475 -> [w491 _]
                  frame "Sensor", Default {
                    n176 = Format Into String(format string="SELECT * from `instrument` where `channel` ='%s'" ("SQL query"), error in=w509, w491) -> (resulting string=w514:string, error out=w515:errorcluster)  [unwired: 1 in]
                    n177 = call "Main - Database (SubVI).vi"("Enum"=FGV_States."Read", "error in (no error)"=w515, "SQL query"=w514) -> ("error out"=w492:errorcluster, "data"=w513:string[][])  [unwired: 7 in]
                    n178 = Index Array(array=w513, index (row)=0) -> (element=w508:string[])  [unwired: 1 in]
                    n179 = Index Array(array=w508, index #1=6 ("index"), index #2=12 ("index"), index #3=13 ("index"), index #4=14 ("index"), index #5=15 ("index")) -> (element #1=w489:string, element #2=w487:string, element #3=w502:string, element #4=w501:string, element #5=w494:string)
                    n180 = Fract/Exp String To Number(string=w489) -> (number=w488:dbl)  [unwired: 3 in, 1 out]
                    n181 = Fract/Exp String To Number(string=w502) -> (number=w500:dbl)  [unwired: 3 in, 1 out]
                    n182 = Fract/Exp String To Number(string=w501) -> (number=w499:dbl)  [unwired: 3 in, 1 out]
                    n183 = Decimal String To Number(string=w487, default (0L)=u32 0 ("default (0 I32)")) -> (number=w485:u32)  [unwired: 1 in, 1 out]
                    n184 = Spreadsheet String To Array(delimiter (Tab)="||", format string="", spreadsheet string=w494, array type (2D Dbl)=string[] []) -> (array=w496:string[])
                    n185 = local write "Maximum Voltage [V]"(w499) -> ()
                    n186 = local write "Max Capacity [EU]"(w500) -> ()
                    n187 = local write "Offset"(w488) -> ()
                    n188 = for {
                      tunnel: w496 -> [w518] mode=indexing
                      tunnel: [w516] -> w493 mode=indexing
                      n189 = Spreadsheet String To Array(delimiter (Tab)=",,", format string="", spreadsheet string=w518, array type (2D Dbl)=string[] []) -> (array=w516:string[])
                    }
                    n190 = local write "Tab 2"(w485) -> ()
                    n191 = local write "Table Control"(w493) -> ()
                  }
                  frame "Displacement" {
                  }
                }
              }
              frame 4 {
                n192 = Unbundle By Name(w531) -> ("Data"=w529:T7)
                n193 = call "Calibration - Data (FGV).vi"("Action"=FGV_States."Write", "error In"=w525, "Calib"=w529) -> ("error out"=w527:errorcluster, "Calib out"=w528:T7)  [unwired: 7 in]
                n194 = call "Calibration - Slope Trigger (eFGV).vi"("Action"=eFGV_States."Write", "error in"=w527, "Calib"=w528) -> ("error out"=w526:errorcluster)  [unwired: 6 in, 2 out]
              }
              frame 5 {
                n195 = local read "Sensor Port"() -> (w542:T1)
                n196 = case shown="\"TD 1\"..\"TD 12\"" w542 {
                  selector: w542 -> [_ w549 w557]
                  tunnel: w541 -> [w547 w555 w563]
                  tunnel: [w547 w555 w563] -> w538
                  tunnel: ["" ("String") w552 w560] -> w540
                  tunnel: ["" ("String") w551 w559] -> w539
                  frame "Please Select", Default {
                  }
                  frame "TD 1".."TD 12" {
                    n197 = Unbundle By Name(w555) -> ("Data.TD Name"=w554:string[], "Data.TD Unit"=w553:string[])  [unwired: 1 out]
                    n198 = Subtract(x=w549, y=9) -> (x-y=w550:i32)
                    n199 = Index Array(array=w554, index=w550) -> (element=w552:string)
                    n200 = Index Array(array=w553, index=w550) -> (element=w551:string)
                  }
                  frame "LC 1".."LC 8" {
                    n201 = Unbundle By Name(w563) -> ("Data.LC Name"=w562:string[], "Data.LC Unit"=w561:string[])
                    n202 = Subtract(x=w557, y=1) -> (x-y=w556:i32)
                    n203 = Index Array(array=w562, index=w556) -> (element=w560:string)
                    n204 = Index Array(array=w561, index=w556) -> (element=w559:string)
                  }
                }
                n205 = local write "Unit"(w539) -> ()
                n206 = local write "Sensor Name"(w540) -> ()
                n207 = local read "Motor"() -> (w534:T2)
                n208 = Unbundle By Name(w538) -> ("Data.Disp M"=w536:dbl[], "Data.Disp Unit"=w535:string[])
                n209 = Decrement(x=w534) -> (x-1=w537:T2)
                n210 = Index Array(array=w536, index=w537) -> (element=w532:dbl)
                n211 = Index Array(array=w535, index=w537) -> (element=w533:string)
                n212 = local write "Disp M"(w532) -> ()
                n213 = local write "Unit Disp"(w533) -> ()
              }
              frame 3 {
                n214 = case shown="\"Direct Factor\", Default" "Tab 2" {
                  tunnel: ["Offset" w633] -> w575
                  tunnel: [w629 w634] -> w576
                  frame "Direct Factor", Default {
                    n215 = Multiply(x=1.0, y="Max Capacity [EU]") -> (x*y=w622:dbl)
                    n216 = Less?(x="Maximum Voltage [V]", y=1.0) -> (x < y?=w625:bool)
                    n217 = Select(t=w622, s=w625, f="Max Capacity [EU]") -> (s? t:f=w626:dbl)
                    n218 = Divide(x=w626, y="Maximum Voltage [V]") -> (x/y=w629:dbl)
                  }
                  frame "Multiple Point" {
                    n219 = Fract/Exp String To Number(string="Table Control") -> (number=w637:dbl[][])  [unwired: 3 in, 1 out]
                    n220 = Index Array(array=w637, index (col)=0 ("disabled index (col)")) -> (element=w631:dbl[])  [unwired: 1 in]
                    n221 = Index Array(array=w637, index (col)=1 ("disabled index (col)")) -> (element=w632:dbl[])  [unwired: 1 in]
                    n222 = call <vilib>:"Linear Fit.vi"("Y"=w632, "X"=w631) -> ("slope"=w634:dbl, "intercept"=w633:dbl)  [unwired: 9 in, 3 out]
                  }
                }
                n223 = local read "Sensor Name"() -> (w568:string)
                n224 = local read "Sensor Port"() -> (w572:T1)
                n225 = local read "Unit"() -> (w569:string)
                n226 = case shown="\"LC 1\"..\"LC 8\"" w572 {
                  selector: w572 -> [_ w595 w604]
                  tunnel: w576 -> [w581 w585 w613]
                  tunnel: w575 -> [w580 w584 w612]
                  tunnel: w565 -> [w583 w601 w620]
                  tunnel: [w583 w600 w619] -> w564
                  tunnel: w571 -> [w582 w592 w618]
                  tunnel: [w582 w592 w618] -> w570
                  tunnel: w569 -> [_ w591 w611]
                  tunnel: w568 -> [_ w587 w610]
                  tunnel: [w581 w585 w613] -> w567
                  tunnel: [w580 w584 w612] -> w566
                  frame "Please Select", Default {
                  }
                  frame "LC 1".."LC 8" {
                    n227 = Unbundle By Name(w601) -> ("Data.LC MC"=w596:dbl[], "Data.LC Unit"=w593:string[], "Data.LC Name"=w589:string[])
                    n228 = Decrement(x=w595) -> (x-1=w588:T1)
                    n229 = Multiply(x=w588, y=2) -> (x*y=w598:i32)
                    n230 = Increment(x=w598) -> (x+1=w597:i32)
                    n231 = Replace Array Subset(array=w596, new element #1=w585, index #1=w598, new element #2=w584, index #2=w597) -> (w594:dbl[])
                    n232 = Replace Array Subset(array=w593, new element=w591, index=w588) -> (w590:string[])
                    n233 = Replace Array Subset(array=w589, new element=w587, index=w588) -> (w586:string[])
                    n234 = Bundle By Name(cluster=w601, "Data.LC MC"=w594, "Data.LC Unit"=w590, "Data.LC Name"=w586) -> (w600:T6)
                  }
                  frame "TD 1".."TD 12" {
                    n235 = Unbundle By Name(w620) -> ("Data.TD MC"=w614:dbl[], "Data.TD Unit"=w609:string[], "Data.TD Name"=w608:string[])
                    n236 = Subtract(x=w604, y=9) -> (x-y=w603:i32)
                    n237 = Multiply(x=w603, y=2) -> (x*y=w616:i32)
                    n238 = Increment(x=w616) -> (x+1=w615:i32)
                    n239 = Replace Array Subset(array=w614, new element #1=w613, index #1=w616, new element #2=w612, index #2=w615) -> (w605:dbl[])
                    n240 = Replace Array Subset(array=w609, new element=w611, index=w603) -> (w607:string[])
                    n241 = Replace Array Subset(array=w608, new element=w610, index=w603) -> (w606:string[])
                    n242 = Bundle By Name(cluster=w620, "Data.TD MC"=w605, "Data.TD Unit"=w607, "Data.TD Name"=w606) -> (w619:T6)
                  }
                }
                n243 = Number To Fractional String(number=w567) -> (F-format string=w574:string)  [unwired: 3 in]
                n244 = Number To Fractional String(number=w566) -> (F-format string=w573:string)  [unwired: 3 in]
                n245 = Bundle By Name(cluster=w564, "Slope"=w574, "Intercept"=w573) -> (w577:T6)
              }
              frame 0 {
                n246 = Unbundle By Name(w639) -> ("Data.Disp M"=w645:dbl[], "Data.Motor Pulse"=w646:u64)
                n247 = local read "Motor"() -> (w643:T2)
                n248 = To Double Precision Float(number=w646) -> (double precision float=w647:dbl)
                n249 = Decrement(x=w643) -> (x-1=w642:T2)
                n250 = Divide(x=w647, y="Displacement") -> (x/y=w641:dbl)
                "Disp M" <- w641
                n251 = Replace Array Subset(array=w645, new element=w641, index=w642) -> (w638:dbl[])
                n252 = Bundle By Name(cluster=w639, "Data.Disp M"=w638) -> (w640:T6)
              }
              frame 6 {
              }
              frame 3 {
              }
              frame 7 {
                n253 = local read "Motor"() -> (w658:T2)
                n254 = case shown="Default" w658 {
                  selector: w658 -> [w662 _]
                  tunnel: w660 -> [w666 w668]
                  tunnel: [w667 w668] -> w659
                  frame Default {
                    n255 = Bundle By Name(cluster=T10 {"Zero"=TRUE, "Machine Name"=enum."Please Select"} ("Zeroing"), "Machine Name"=w662) -> (w664:T10)
                    n256 = call "Communication - Displacement Zeroing (eFGV).vi"("Action"=eFGV_States."Write", "error in"=w666, "Zeroing"=w664) -> ("error out"=w667:errorcluster)  [unwired: 6 in, 2 out]
                  }
                  frame "Please Select" {
                  }
                }
              }
            }
          }
          frame Error {
            n257 = call <vilib>:"Clear Errors.vi"("error in (no error)"=w673) -> ("error out"=w672:errorcluster)  [unwired: 5 in, 1 out]
            n258 = Wait (ms)(milliseconds to wait=u32 100) -> ()  [unwired: 1 out]
          }
        }
      }
      "error out" <- w4
    }
    frame Enabled {
    }
  }
